vi "Write Calibration config to file.vi"(8 "error in (no error)":errorcluster, 10 "configuration file path":path, 11 "Calibration config.":T1) -> (0 "error out":errorcluster)   [LabVIEW 2020]
uses:
  Typedefs/Calibration config.ctl
  Typedefs/Objective Config.ctl
  Typedefs/Prechirper Cal Config.ctl
  Typedefs/PreChirper constants.ctl
  <vilib>/Utility/config.llb/Write Key (String).vi
  <vilib>/Utility/config.llb/Write Key (Double).vi
  <vilib>/Utility/config.llb/Write Key (Boolean).vi
  <vilib>/Utility/config.llb/Write Key (I32).vi
  <vilib>/Utility/config.llb/NI_LVConfig.lvlib
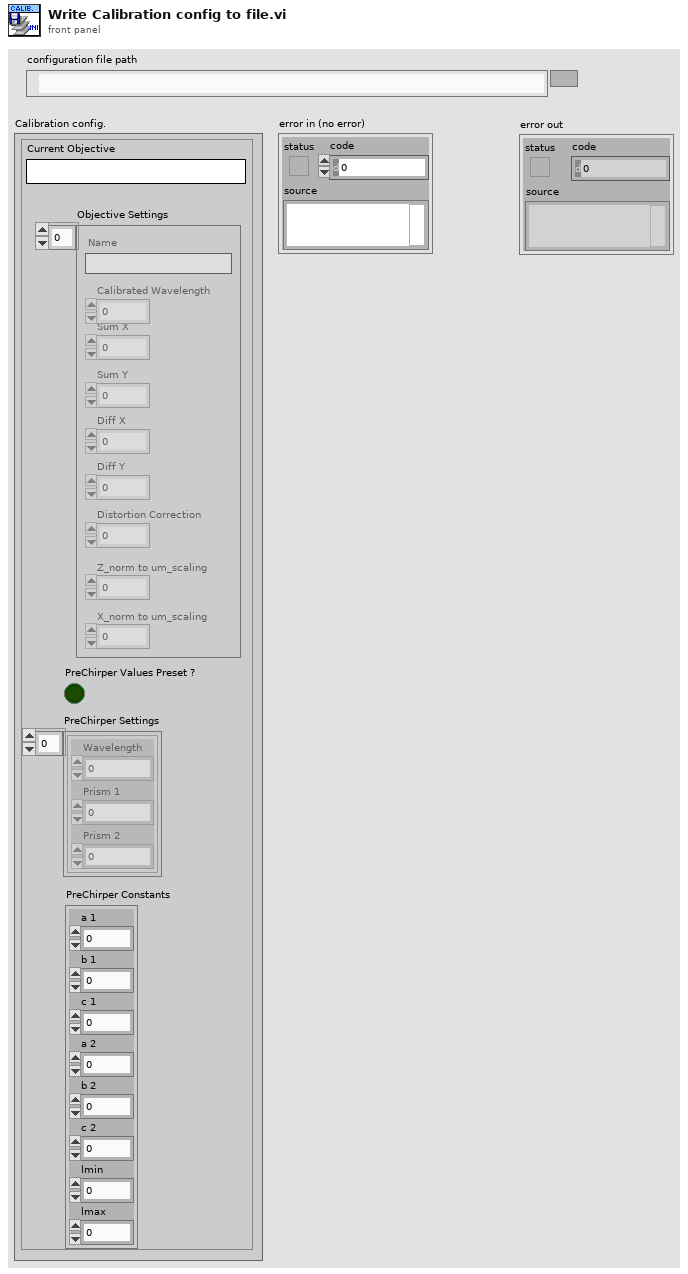
[diagram p1: front panel]
types:
  T1 = typedef "Calibration config.ctl" = cluster{"Current Objective":string, "Objective Settings":T2[], "PreChirper Values Preset ?":bool, "PreChirper Settings":T3[], "PreChirper Constants":T4}
  T2 = typedef "Objective Config.ctl" = cluster{"Name":string, "Sum X":dbl, "Sum Y":dbl, "Diff X":dbl, "Diff Y":dbl, "Distortion Correction":dbl, "Z_norm to um_scaling":dbl, "X_norm to um_scaling":dbl, "Calibrated Wavelength":dbl}
  T3 = typedef "Prechirper Cal Config.ctl" = cluster{"Wavelength":i32, "Prism 1":i32, "Prism 2":i32}
  T4 = typedef "PreChirper constants.ctl" = cluster{"a 1":i32, "b 1":i32, "c 1":i32, "a 2":i32, "b 2":i32, "c 2":i32, "lmin":i32, "lmax":i32}
  T5 = typedef "NI_LVConfig.lvlib/Config Data RefNum.ctl" = refnum<k1>
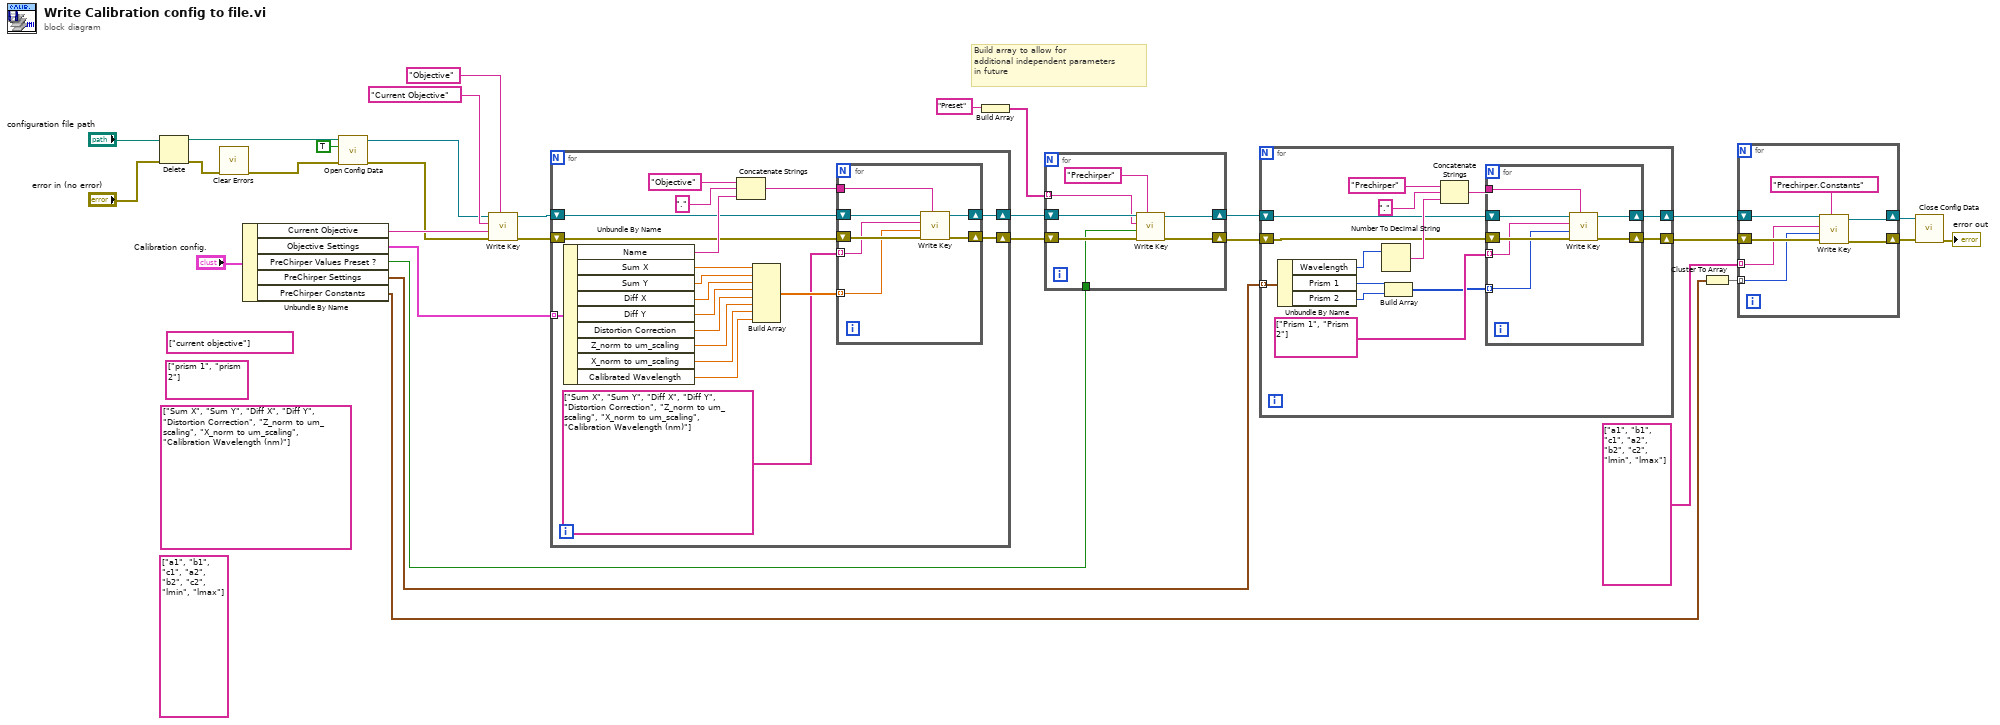
[diagram p0: block diagram]
diagram:
  (unwired) string[] ["a1", "b1", "c1", "a2", "b2", "c2", "lmin", "lmax"]
  (unwired) string[] ["Sum X", "Sum Y", "Diff X", "Diff Y", "Distortion Correction", "Z_norm to um_scaling", "X_norm to um_scaling", "Calibration Wavelength (nm)"] ("array (last n elements first)")
  (unwired) string[] ["prism 1", "prism 2"]
  (unwired) string[] ["current objective"]
  # "Build array to allow for \nadditional independent parameters\nin future"
  n1 = Delete(path (use dialog)="configuration file path", error in="error in (no error)") -> (deleted path=w19:path, error out=w2:errorcluster)  [unwired: 3 in, 1 out]
  n2 = call <vilib>:"Clear Errors.vi"("error in (no error)"=w2) -> ("error out"=w1:errorcluster)  [unwired: 5 in, 1 out]
  n3 = Unbundle By Name("Calibration config.") -> ("Current Objective"=w29:string, "Objective Settings"=w24:T2[], "PreChirper Values Preset ?"=w15:bool, "PreChirper Settings"=w16:T3[], "PreChirper Constants"=w10:T4)
  n4 = call <vilib>:"Open Config Data.vi"("error in (no error)"=w1, "create file if necessary (T)"=TRUE, "configuration file path"=w19) -> ("error out"=w26:errorcluster, "refnum"=w27:T5)  [unwired: 6 in, 1 out]
  n5 = call-poly <vilib>:"Write Key.vi"("section"="Objective", "error in (no error)"=w26, "value"=w29, "key"="Current Objective", "refnum"=w27) -> ("error out"=w23:errorcluster, "refnum out"=w25:T5)  [unwired: 4 in, 1 out]
  n6 = for {
    tunnel: w24 -> [w50] mode=indexing
    shift-right: [w34] -> w17
    shift-left: w25 -> [w36]
    shift-right: [w32] -> w18
    shift-left: w23 -> [w33]
    n7 = Unbundle By Name(w50) -> ("Name"=w47:string, "Sum X"=w46:dbl, "Sum Y"=w45:dbl, "Diff X"=w44:dbl, "Diff Y"=w43:dbl, "Distortion Correction"=w42:dbl, "Z_norm to um_scaling"=w41:dbl, "X_norm to um_scaling"=w40:dbl, "Calibrated Wavelength"=w39:dbl)
    n8 = Concatenate Strings("Objective" ("section"), "." ("string"), w47) -> (w35:string)
    n9 = Build Array(w46, w45, w44, w43, w42, w41, w40, w39) -> (w38:dbl[])
    n10 = for {
      tunnel: w38 -> [w54] mode=indexing
      tunnel: string[] ["Sum X", "Sum Y", "Diff X", "Diff Y", "Distortion Correction", "Z_norm to um_scaling", "X_norm to um_scaling", "Calibration Wavelength (nm)"] ("array (last n elements first)") -> [w55] mode=indexing
      tunnel: w35 -> [w53]
      shift-right: [w52] -> w34
      shift-left: w36 -> [w57]
      shift-right: [w51] -> w32
      shift-left: w33 -> [w56]
      n11 = call-poly <vilib>:"Write Key.vi"("section"=w53, "error in (no error)"=w56, "value"=w54, "key"=w55, "refnum"=w57) -> ("error out"=w51:errorcluster, "refnum out"=w52:T5)  [unwired: 4 in, 1 out]
    }
  }
  n12 = Build Array("Preset" ("key")) -> (w4:string[])
  n13 = for {
    shift-right: [w63] -> w14
    shift-left: w18 -> [w64]
    shift-right: [w61] -> w13
    shift-left: w17 -> [w62]
    tunnel: w15 -> [w59]
    tunnel: w4 -> [w58] mode=indexing
    n14 = call-poly <vilib>:"Write Key.vi"("section"="Prechirper", "error in (no error)"=w64, "value"=w59, "key"=w58, "refnum"=w62) -> ("error out"=w63:errorcluster, "refnum out"=w61:T5)  [unwired: 4 in, 1 out]
  }
  n15 = for {
    tunnel: w16 -> [w76] mode=indexing
    shift-right: [w70] -> w12
    shift-left: w14 -> [w72]
    shift-right: [w71] -> w11
    shift-left: w13 -> [w73]
    n16 = Unbundle By Name(w76) -> ("Wavelength"=w75:i32, "Prism 1"=w67:i32, "Prism 2"=w66:i32)
    n17 = Number To Decimal String(number=w75) -> (decimal integer string=w74:string)  [unwired: 1 in]
    n18 = Build Array(w67, w66) -> (w65:i32[])
    n19 = Concatenate Strings("Prechirper" ("section"), "." ("string"), w74) -> (w69:string)
    n20 = for {
      tunnel: w65 -> [w82] mode=indexing
      tunnel: string[] ["Prism 1", "Prism 2"] -> [w83] mode=indexing
      tunnel: w69 -> [w81]
      shift-right: [w80] -> w71
      shift-left: w73 -> [w85]
      shift-right: [w79] -> w70
      shift-left: w72 -> [w84]
      n21 = call-poly <vilib>:"Write Key.vi"("section"=w81, "error in (no error)"=w84, "value"=w82, "key"=w83, "refnum"=w85) -> ("error out"=w79:errorcluster, "refnum out"=w80:T5)  [unwired: 4 in, 1 out]
    }
  }
  n22 = Cluster To Array(cluster=w10) -> (array=w8:i32[])
  n23 = for {
    shift-right: [w87] -> w7
    shift-left: w12 -> [w92]
    shift-right: [w86] -> w6
    shift-left: w11 -> [w91]
    tunnel: string[] ["a1", "b1", "c1", "a2", "b2", "c2", "lmin", "lmax"] -> [w88] mode=indexing
    tunnel: w8 -> [w89] mode=indexing
    n24 = call-poly <vilib>:"Write Key.vi"("section"="Prechirper.Constants", "error in (no error)"=w92, "value"=w89, "key"=w88, "refnum"=w91) -> ("error out"=w87:errorcluster, "refnum out"=w86:T5)  [unwired: 4 in, 1 out]
  }
  n25 = call <vilib>:"Close Config Data.vi"("error in (no error)"=w7, "refnum"=w6) -> ("error out"=→"error out":errorcluster)  [unwired: 8 in, 1 out]
